vi "controller.vi"(0 "position":dbl, 1 "pos ref":dbl, 3 "velocity":dbl, 4 "vel ref":dbl, 9 "K2":dbl, 10 "K1":dbl) -> (15 "duty out":dbl)   [LabVIEW 2019]
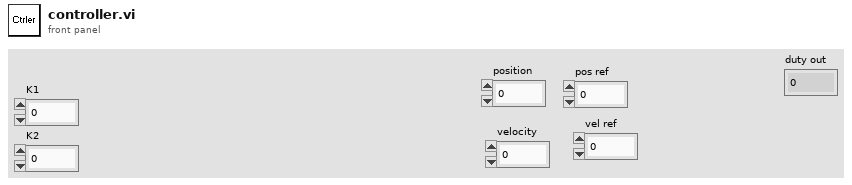
[diagram p1: front panel]
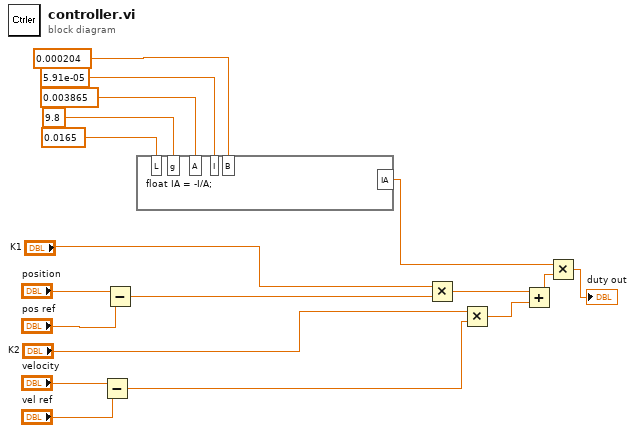
[diagram p0: block diagram]
diagram:
  n1 = Subtract(x="velocity", y="vel ref") -> (x-y=w11:dbl)
  n2 = Subtract(x="position", y="pos ref") -> (x-y=w12:dbl)
  n3 = formula code="float IA = -I/A;"("L"=0.0165 ("input variable"), "g"=9.8 ("input variable 2"), "A"=0.003865 ("input variable 3"), "I"=5.91e-05 ("input variable 4"), "B"=0.000204 ("input variable 5")) -> ("IA"=w3:dbl)
  n4 = Multiply(x="K1", y=w12) -> (x*y=w15:dbl)
  n5 = Multiply(x="K2", y=w11) -> (x*y=w14:dbl)
  n6 = Add(x=w15, y=w14) -> (x+y=w10:dbl)
  n7 = Multiply(x=w3, y=w10) -> (x*y=→"duty out":dbl)
